vi "Disarm.vi"(8 "error in (no error)":errorcluster, 9 "Request type":T1=enum."User command", 11 "DAQmx Digitizer in":refnum<class "DAQmx Synthesizer.lvclass">) -> (0 "error out":errorcluster, 2 "Armed":bool, 3 "DAQmx Digitizer out":refnum<class "DAQmx Synthesizer.lvclass">)   [LabVIEW 2021, in "DAQmx Synthesizer.lvclass"]
uses:
  DAQmx Synthesizer.lvclass
  LabActor/Controllers/Process Controller/Request type.ctl
  DAQmx Synthesizer.lvclass/DAQmx Synthesizer.ctl
  DAQmx Digitizer/DAQmx Digitizer.lvclass
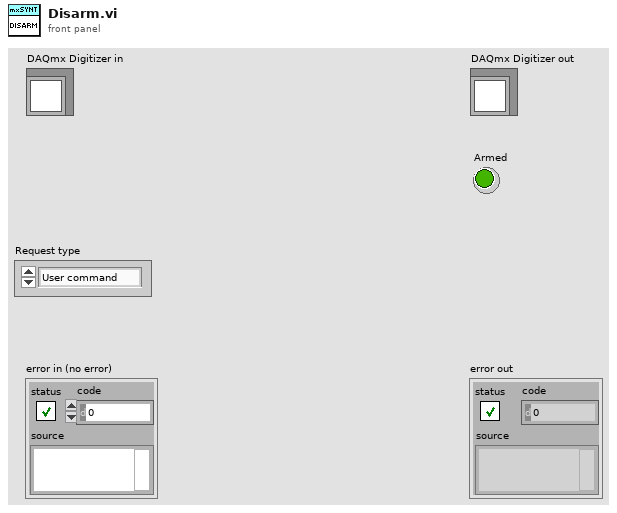
[diagram p1: front panel]
types:
  T1 = typedef "Request type.ctl" = enum16{"Process complete", "User command", "Auto-restart", "Error"}
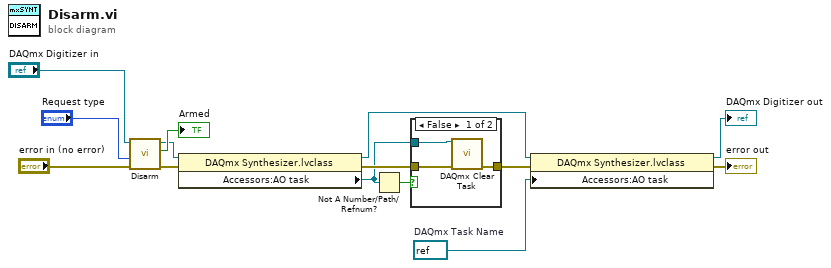
[diagram p0: block diagram]
diagram:
  w4 = refnum<k21> refnum  # DAQmx Task Name
  n1 = call-parent "Disarm.vi"("error in (no error)"="error in (no error)", "Request type"="Request type", "DAQmx Digitizer in"="DAQmx Digitizer in") -> ("error out"=w1:errorcluster, "Armed"=→"Armed":bool, "DAQmx Digitizer out"=w5:refnum<class "DAQmx Synthesizer.lvclass">)  [unwired: 6 in]
  n2 = property class="DAQmx Synthesizer.lvclass"(reference=w5, error in=w1) -> (reference out=w7:refnum<class "DAQmx Synthesizer.lvclass">, error out=w9:errorcluster, "Accessors:AO task"=w6:refnum<k21>)
  n3 = Not A Number/Path/Refnum?(number/path/refnum=w6) -> (NaN/Path/Refnum?=w10:bool)
  n4 = case shown="False" w10 {
    tunnel: w6 -> [w17 _]
    tunnel: w9 -> [w16 w18]
    tunnel: [w15 w18] -> w8
    frame False {
      n5 = call <vilib>:"DAQmx Clear Task.vi"("task in"=w17, "error in"=w16) -> ("error out"=w15:errorcluster)  [unwired: 13 out]
    }
    frame True {
    }
  }
  n6 = property class="DAQmx Synthesizer.lvclass"(reference=w7, error in=w8, "Accessors:AO task"=w4) -> (reference out=→"DAQmx Digitizer out":refnum<class "DAQmx Synthesizer.lvclass">, error out=→"error out":errorcluster)
